vi "Make Versioned Name.vi"() -> (1 "LV Version":string, 3 "versioned name":string)   [LabVIEW 2020, in "LMH-LINX.lvlib"]
uses:
  LMH-LINX.lvlib
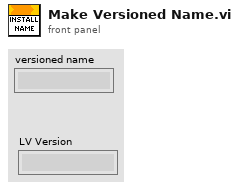
[diagram p1: front panel]
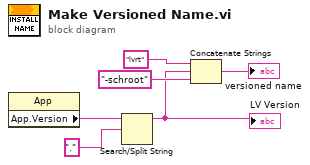
[diagram p0: block diagram]
diagram:
  n1 = property class="App"() -> ("App.Version"=w6:string)  [unwired: 2 in, 2 out]
  n2 = Search/Split String(string=w6, search string/char (-)=".") -> (substring before match=w1:string)  [unwired: 1 in, 2 out]
  "LV Version" <- w1
  n3 = Concatenate Strings("lvrt" ("search string/char (-)"), w1, "-schroot" ("search string/char (-)")) -> (→"versioned name":string)
